vi "Actor Core.vi"(8 "error in":errorcluster, 11 "Nested in":refnum<class "Dinero.lvclass">) -> (0 "error out":errorcluster, 3 "Actor out":refnum<class "Actor.lvclass">)   [LabVIEW 2020, in "Dinero.lvlib" / "Dinero.lvclass"]
doc: "(<B>Filename</B>: Actor Framework.lvlib:Actor.lvclass:Actor Core.vi)\n\nReceives messages to the actor, reacts to them, and initiates any error handling that may shut the actor down.\n\nDescendant classes may override this VI to append parallel tasks for the actor to complete while it handles messages. Overrides use the Call Parent Method node."
uses:
  Dinero.lvclass
  C:/Program Files (x86)/National Instruments/LabVIEW 2020/vi.lib/ActorFramework/Actor/Actor.lvclass
  <vilib>/ActorFramework/Actor/Actor.lvclass
  <vilib>/ActorFramework/Actor/Actor.lvclass/Actor.ctl
  <vilib>/ActorFramework/Message Enqueuer/Message Enqueuer.lvclass/Message Enqueuer.ctl
  Dinero.lvclass/Dinero.ctl
  Dinero Messages/Aumento Credito Msg/Aumento Credito Msg.lvclass/Aumento Credito Msg.ctl
  <vilib>/ActorFramework/Message Enqueuer/Init from Existing Queue.vi
  <vilib>/ActorFramework/Message Enqueuer/Enqueue.vi
  <vilib>/ActorFramework/Stop Msg/Stop Msg.lvclass
  C:/Program Files (x86)/National Instruments/LabVIEW 2020/vi.lib/ActorFramework/Message/Message.lvclass
  Dinero Messages/Aumento Credito Msg/Aumento Credito Msg.lvclass
  <vilib>/ActorFramework/Message Priority Queue/Priority Enqueue.vi
  <vilib>/ActorFramework/Message Enqueuer/Message Enqueuer.lvclass
panel:
  out "Cambio":dbl
  out "Credito":dbl
  in  "200 $":bool
  in  "50 $":bool
  in  "100 $":bool
  in  "20 $":bool
  in  "10 $":bool
  in  "5 $":bool
  in  "2 $":bool
  in  "1 $":bool
  # "MONEDAS"
  # "BILLETES"
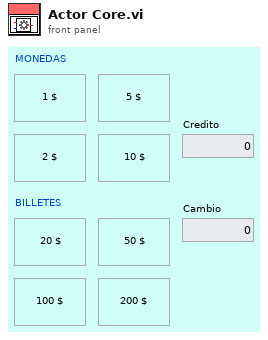
[diagram p1: front panel]
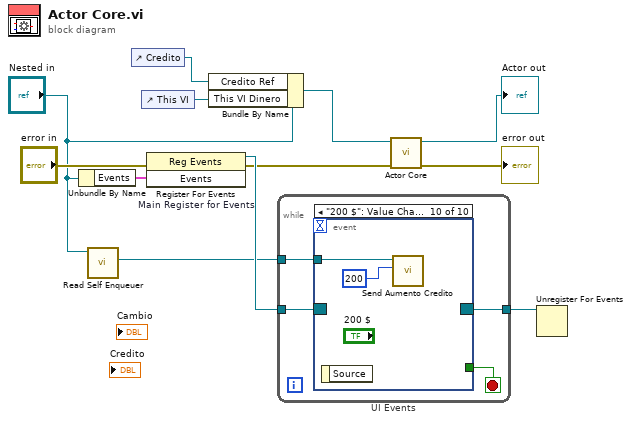
[diagram p0: block diagram]
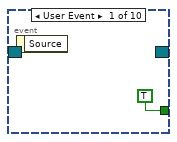
[diagram p2: hidden frame]
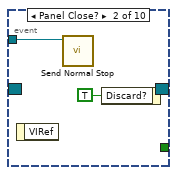
[diagram p3: hidden frame]
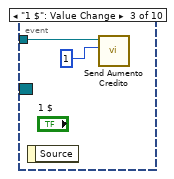
[diagram p4: hidden frame]
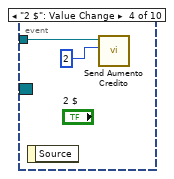
[diagram p5: hidden frame]
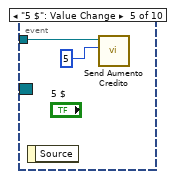
[diagram p6: hidden frame]
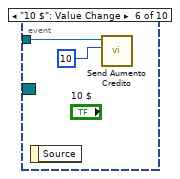
[diagram p7: hidden frame]
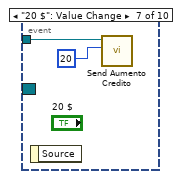
[diagram p8: hidden frame]
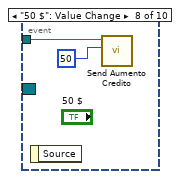
[diagram p9: hidden frame]
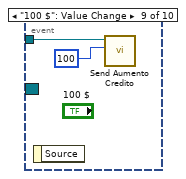
[diagram p10: hidden frame]
diagram:
  n1 = Unbundle By Name("Nested in") -> ("Events"=w9:cluster{"Stop":refnum<user-event>})
  n2 = call <vilib>:"Read Self Enqueuer.vi"("Actor"="Nested in") -> ("Self Enqueuer"=w7:refnum<class "Message Enqueuer.lvclass">)  [unwired: 10 in]
  n3 = control-ref of="Credito"() -> (w1:refnum<vi>)
  n4 = control-ref of="This VI"() -> (w2:refnum<vi>)
  n5 = register-events "Main Register for Events"(error in="error in", w9) -> (reference out=w10:refnum<event-registration>, error out=w5:errorcluster)  [unwired: 1 in]
  n6 = Bundle By Name(cluster="Nested in", "Credito Ref"=w1, "This VI Dinero"=w2) -> (w3:refnum<class "Dinero.lvclass">)
  n7 = while {
    tunnel: w10 -> [w16]
    tunnel: [w14] -> w8
    tunnel: w7 -> [w13]
    stop <- w15 stop-if-true
    n8 = event "UI Events" shown="[9] \"200 $\": Value Change" {
      selector: w16 -> [_ _ _ _ _ _ _ _ _ _]
      dyn-events: [_ _ _ _ _ _ _ _ _ _] -> w14
      timeout: _ -> [_ _ _ _ _ _ _ _ _ _]
      tunnel: [TRUE _ _ _ _ _ _ _ _ _] -> w15
      tunnel: w13 -> [_ w18 w21 w23 w25 w27 w29 w31 w33 w35]
      event User Event {
        n9 = event-data() -> ()  [unwired: 1 in, 1 out]
      }
      event Panel Close? {
        n10 = event-data() -> ()  [unwired: 1 in, 1 out]
        n11 = call <vilib>:"Send Normal Stop.vi"("Message Enqueuer"=w18) -> ()  [unwired: 10 in, 1 out]
        n12 = event-data("Discard?"=TRUE) -> ()  [unwired: 1 in, 1 out]
      }
      event "1 $": Value Change {
        n13 = event-data() -> ()  [unwired: 1 in, 1 out]
        n14 = call "Send Aumento Credito.vi"("Dinero"=1, "Message Enqueuer"=w21) -> ()  [unwired: 8 in, 2 out]
      }
      event "2 $": Value Change {
        n15 = event-data() -> ()  [unwired: 1 in, 1 out]
        n16 = call "Send Aumento Credito.vi"("Dinero"=2, "Message Enqueuer"=w23) -> ()  [unwired: 8 in, 2 out]
      }
      event "5 $": Value Change {
        n17 = event-data() -> ()  [unwired: 1 in, 1 out]
        n18 = call "Send Aumento Credito.vi"("Dinero"=5, "Message Enqueuer"=w25) -> ()  [unwired: 8 in, 2 out]
      }
      event "10 $": Value Change {
        n19 = event-data() -> ()  [unwired: 1 in, 1 out]
        n20 = call "Send Aumento Credito.vi"("Dinero"=10, "Message Enqueuer"=w27) -> ()  [unwired: 8 in, 2 out]
      }
      event "20 $": Value Change {
        n21 = event-data() -> ()  [unwired: 1 in, 1 out]
        n22 = call "Send Aumento Credito.vi"("Dinero"=20, "Message Enqueuer"=w29) -> ()  [unwired: 8 in, 2 out]
      }
      event "50 $": Value Change {
        n23 = event-data() -> ()  [unwired: 1 in, 1 out]
        n24 = call "Send Aumento Credito.vi"("Dinero"=50, "Message Enqueuer"=w31) -> ()  [unwired: 8 in, 2 out]
      }
      event "100 $": Value Change {
        n25 = event-data() -> ()  [unwired: 1 in, 1 out]
        n26 = call "Send Aumento Credito.vi"("Dinero"=100, "Message Enqueuer"=w33) -> ()  [unwired: 8 in, 2 out]
      }
      event "200 $": Value Change {
        n27 = event-data() -> ()  [unwired: 1 in, 1 out]
        n28 = call "Send Aumento Credito.vi"("Dinero"=200, "Message Enqueuer"=w35) -> ()  [unwired: 8 in, 2 out]
      }
    }
  }
  n29 = call-parent "Actor Core.vi"("error in"=w5, "Actor in"=w3) -> ("error out"=→"error out":errorcluster, "Actor out"=→"Actor out":refnum<class "Actor.lvclass">)  [unwired: 8 in]
  n30 = Unregister For Events(event registration refnum=w8) -> ()  [unwired: 1 in, 1 out]
